vi "Non Callback Test.vi"() -> ()   [LabVIEW 2011]
uses:
  <vilib>/Platform/TimedLoop/XDataNode/timing_clust.ctl
  <vilib>/Platform/TimedLoop/XDataNode/nitl_modes.ctl
  <vilib>/Platform/TimedLoop/XDataNode/wakeup.ctl
  <vilib>/vision/Image Controls.llb/IMAQ Image.ctl
  C:/Users/Behavior Room/Desktop/Kinect Mouse/DepthSense/FunctionPointerProxy/FunctionPointerProxy/bin/Release/FunctionPointerProxy.dll
  FunctionPointerProxy/FunctionPointerProxy/bin/Release/FunctionPointerProxy.dll
  DepthSense Global Status.vi
  <vilib>/Platform/TimedLoop/XDataNode/XDataNode.xnode
  <userlib>/libOptrima-2-3/libOptrima-2-3.lvlib
  <vilib>/Platform/TimedLoop/XDataNode/XDNodeRunTimeDep.lvlib
  Program Files (x86)/SoftKinetic/OptrimaSDK/lib/libOptrima-2-3.dll
panel:
  out "DepthSense Status":T1={"Camera Version"="", "Image Height"=0, "Image Width"=0, "Minimum Framerate"=0, "Maximum Framerate"=0, "Framerate"=60, "Close Mode"=FALSE, "Denoising"=FALSE, "Leakage Algorithm"=FALSE, "Anti-Aliasing"=FALSE, "Camera Status"=-2, "API Version"="", "Light Intensity"=100, "Confidence Threshold"=100}
  out "Image":T2(plugin-control)
  in  "stop":bool
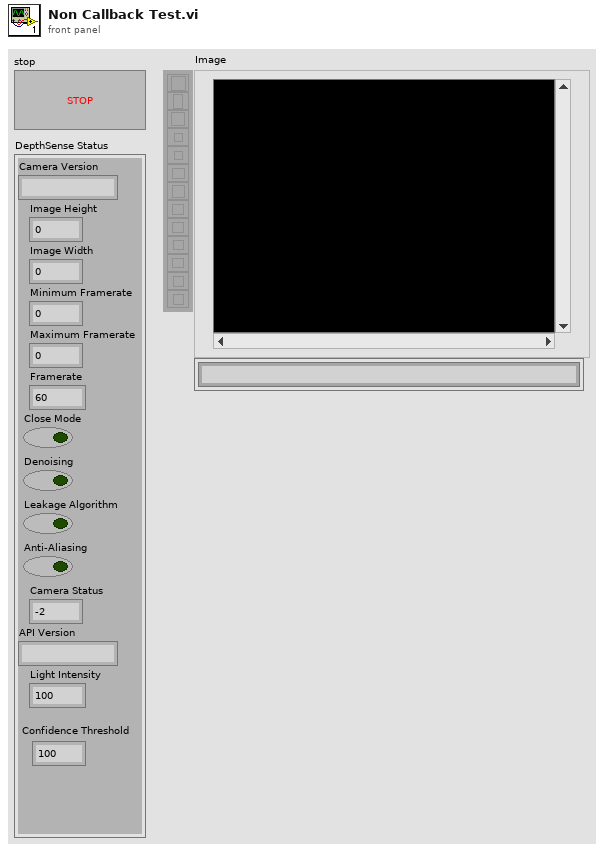
[diagram p1: front panel]
types:
  T1 = cluster{"Camera Version":string, "Image Height":i32, "Image Width":i32, "Minimum Framerate":i32, "Maximum Framerate":i32, "Framerate":i32, "Close Mode":bool, "Denoising":bool, "Leakage Algorithm":bool, "Anti-Aliasing":bool, "Camera Status":i32, "API Version":string, "Light Intensity":i32, "Confidence Threshold":u16}
  T2 = typedef "IMAQ Image.ctl" = refnum<image>
  T3 = typedef "t_CallbackReferences.ctl" = cluster{"LV event callback ":refnum<k27>, "Proxy instance":refnum<k24>, "(*f)(...)":i32}
  T4 = typedef "XDNodeRunTimeDep.lvlib/timing_clust.ctl" = cluster{"Expected End [f-1]":u64, "Actual End [f-1]":u64, "Finished Late? [f-1]":bool, "Expected End [i-1]":u64, "Actual End [i-1]":u64, "Finished Late? [i-1]":bool, "Expected Start [i]":u64, "Actual Start [i]":u64, "Expected Start [f]":u64, "Actual Start [f]":u64, "Source Name":string, "Structure Name":string, "Period":i64, "Deadline":i64, "Offset":i64, "Start":i64, "Priority":i32, "Timeout":i32, "Mode":T5, "Wakeup Reason":T6, "Error":errorcluster, "Source Type":string, "Secondary Source Type":string, "Global End Time":u64, "Global Start Time":u64, "Frame Duration":u64, "Iteration Duration":u64, "Assigned CPU":i32, "I/O Scan Engine Mode":u32}
  T5 = typedef "XDNodeRunTimeDep.lvlib/nitl_modes.ctl" = enum32{"No Change", "Process missed periods, maintain original phase", "Discard missed periods, maintain original phase", "Process missed periods, ignore original phase", "Discard missed periods, ignore original phase"}
  T6 = typedef "XDNodeRunTimeDep.lvlib/wakeup.ctl" = enum32{"Normal", "Aborted", "Asynchronous wakeup", "Timing source error", "Timed loop error", "Timeout"}
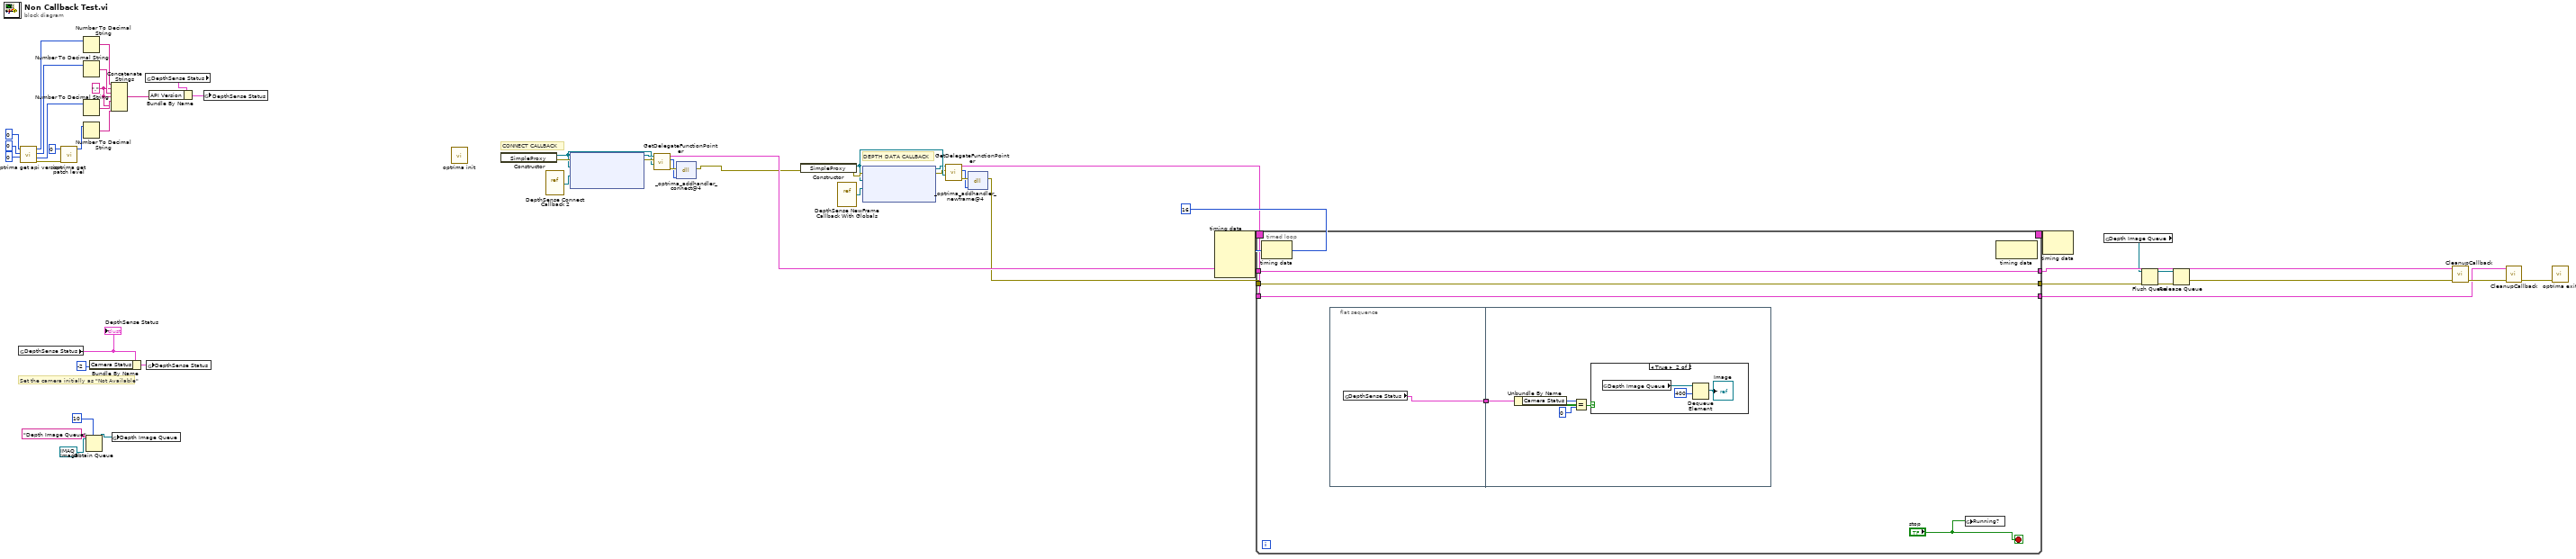
[diagram p0: block diagram]
diagram:
  w41 = "."
  # "Set the camera initially as \"Not Available\""
  # "DEPTH DATA CALLBACK"
  # "CONNECT CALLBACK"
  n1 = global read "DepthSense Global Status.vi" "DepthSense Status"() -> (w6:T1)
  "DepthSense Status" <- w6
  n2 = call <userlib>:"optrima get api version.vi"("minor"=u32 0, "major"=u32 0, "release"=u32 0) -> ("error out"=w54:errorcluster, "minor out"=w51:u32, "major out"=w52:u32, "release out"=w53:u32)  [unwired: 5 in]
  n3 = call <userlib>:"optrima get patch level.vi"("error in (no error)"=w54, "patch"=u32 0) -> ("patch out"=w50:u32)  [unwired: 8 in, 1 out]
  n4 = Number To Decimal String(number=w53) -> (decimal integer string=w49:string)  [unwired: 1 in]
  n5 = Number To Decimal String(number=w52) -> (decimal integer string=w44:string)  [unwired: 1 in]
  n6 = Number To Decimal String(number=w51) -> (decimal integer string=w43:string)  [unwired: 1 in]
  n7 = Number To Decimal String(number=w50) -> (decimal integer string=w42:string)  [unwired: 1 in]
  n8 = Obtain Queue(max queue size (-1, unlimited)=10, name (unnamed)="Depth Image Queue", element data type=T2 refnum ("New Image")) -> (queue out=w23:refnum<queue>)  [unwired: 2 in, 2 out]
  n9 = Bundle By Name(cluster=w6, "Camera Status"=-2) -> (w30:T1)
  n10 = Concatenate Strings(w49, w41, w44, w41, w43, w41, w42) -> (w31:string)
  n11 = global write "DepthSense Global Status.vi" "Depth Image Queue"(w23) -> ()
  n12 = global read "DepthSense Global Status.vi" "DepthSense Status"() -> (w32:T1)
  n13 = global write "DepthSense Global Status.vi" "DepthSense Status"(w30) -> ()
  n14 = Bundle By Name(cluster=w32, "API Version"=w31) -> (w33:T1)
  n15 = global write "DepthSense Global Status.vi" "DepthSense Status"(w33) -> ()
  n16 = call <userlib>:"optrima init.vi"() -> ()  [unwired: 11 in, 1 out]
  n17 = constructor class="SimpleProxy"() -> (reference out=w37:refnum<k24>, error out=w40:errorcluster)  [unwired: 3 in, 1 out]
  n18 = vi-ref "DepthSense Connect Callback 2.vi"() -> ("vi reference"=w22:refnum<vi>)
  n19 = node(w40, w37, w22) -> (w39:refnum<k27>, w38:errorcluster)  [unwired: 2 in]
  n20 = call "GetDelegateFunctionPointer.vi"("target class"=w37, "error in (no error)"=w38, "event callback refnum"=w39) -> ("error out"=w36:errorcluster, "(*f)(...)"=w35:i32, "References"=w34:T3)  [unwired: 6 in]
  n21 = dll-call lib="C:/Program Files (x86)/SoftKinetic/OptrimaSDK/lib/libOptrima-2-3.dll" fn="_optrima_addhandler_connect@4"(error in=w36, "handlerfunc"=w35) -> (error out=w11:errorcluster)  [unwired: 4 in, 1 out]
  n22 = constructor class="SimpleProxy"(error in=w11) -> (reference out=w20:refnum<k24>, error out=w21:errorcluster)  [unwired: 2 in, 1 out]
  n23 = vi-ref "DepthSense NewFrame Callback With Globals.vi"() -> ("vi reference"=w15:refnum<vi>)
  n24 = node(w21, w20, w15) -> (w18:refnum<k27>, w19:errorcluster)  [unwired: 2 in]
  n25 = call "GetDelegateFunctionPointer.vi"("target class"=w20, "error in (no error)"=w19, "event callback refnum"=w18) -> ("error out"=w17:errorcluster, "(*f)(...)"=w16:i32, "References"=w14:T3)  [unwired: 6 in]
  n26 = dll-call lib="C:/Program Files (x86)/SoftKinetic/OptrimaSDK/lib/libOptrima-2-3.dll" fn="_optrima_addhandler_newframe@4"(error in=w17, "handlerfunc"=w16) -> (error out=w12:errorcluster)  [unwired: 4 in, 1 out]
  n27 = node-c288(i64 16 ("Period")) -> (w28:T4)  [unwired: 3 in]
  n28 = timed-loop {
    tunnel: [w59] -> w2
    tunnel: w12 -> [w59]
    tunnel: [w58] -> w8
    tunnel: w34 -> [w58]
    timing: w28 -> [_]
    timing-out: [_] -> w27
    tunnel: w14 -> [w57]
    tunnel: [w57] -> w7
    stop <- "stop" stop-if-true
    n29 = node-c288() -> ()  [unwired: 1 in, 1 out]
    n30 = flat-sequence {
      tunnel: [w60] -> w56
      tunnel: w56 -> [w61]
      frame #0 {
        n31 = global read "DepthSense Global Status.vi" "DepthSense Status"() -> (w60:T1)
      }
      frame #1 {
        n32 = Unbundle By Name(w61) -> ("Camera Status"=w63:i32)
        n33 = Equal?(x=w63, y=0) -> (x = y?=w64:bool)
        n34 = case shown="True" w64 {
          frame False {
          }
          frame True {
            n35 = global read "DepthSense Global Status.vi" "Depth Image Queue"() -> (w67:refnum<queue>)
            n36 = Dequeue Element(queue=w67, timeout in ms (-1)=400) -> (element=→"Image":T2)  [unwired: 1 in, 3 out]
          }
        }
      }
    }
    n37 = global write "DepthSense Global Status.vi" "Running?"("stop") -> ()
    n38 = node-c288() -> ()  [unwired: 1 in, 1 out]
  }
  n39 = node-c288(w27) -> ()  [unwired: 1 out]
  n40 = global read "DepthSense Global Status.vi" "Depth Image Queue"() -> (w3:refnum<queue>)
  n41 = Flush Queue(queue=w3, error in (no error)=w2) -> (queue out=w5:refnum<queue>, error out=w4:errorcluster)  [unwired: 1 out]
  n42 = Release Queue(queue=w5, error in (no error)=w4) -> (error out=w1:errorcluster)  [unwired: 1 in, 2 out]
  n43 = call "CleanupCallback.vi"("error in (no error)"=w1, "References"=w8) -> ("error out"=w9:errorcluster)  [unwired: 9 in]
  n44 = call "CleanupCallback.vi"("error in (no error)"=w9, "References"=w7) -> ("error out"=w10:errorcluster)  [unwired: 9 in]
  n45 = call <userlib>:"optrima exit.vi"("error in (no error)"=w10) -> ()  [unwired: 10 in, 1 out]
